vi "publishSlitWidth.vi"(8 "error in (no error)":errorcluster, 10 "slitPosition":T1, 11 "Monochromator in":refnum<class "Monochromator.lvclass">) -> (0 "error out":errorcluster, 3 "Monochromator out":refnum<class "Monochromator.lvclass">)   [LabVIEW 2016, in "Monochromator.lvclass"]
uses:
  Monochromator.lvclass
  Typedefs/slit.ctl
  Typedefs/SlitType.ctl
  Typedefs/slitWidth.ctl
  Monochromator.lvclass/Monochromator.ctl
  MonoPubSubData/MonoPubSubData.lvclass/MonoPubSubData.ctl
  MonoPubSubData/MonoPubSubData.lvclass
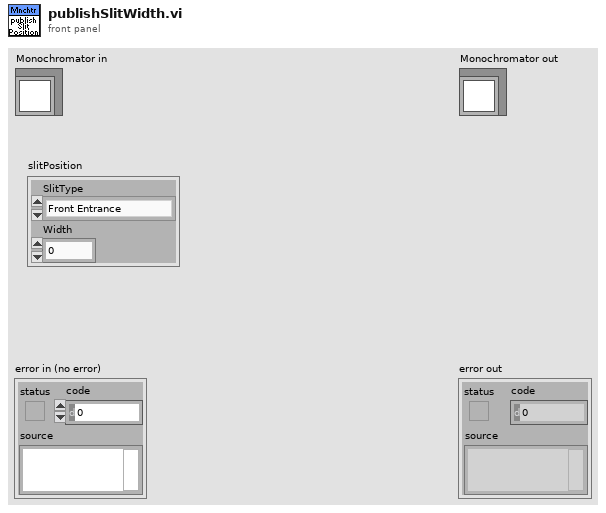
[diagram p1: front panel]
types:
  T1 = typedef "slit.ctl" = cluster{"SlitType":T2, "Width":T3}
  T2 = typedef "SlitType.ctl" = enum16{"Front Entrance", "Side Entrance", "Front Exit", "Side Exit", "First Intermediate", "Second Intermediate"}
  T3 = typedef "slitWidth.ctl" = dbl
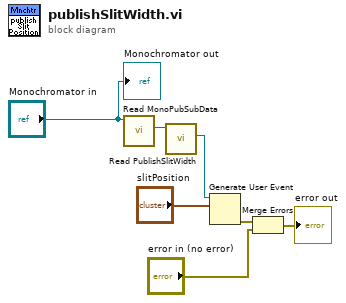
[diagram p0: block diagram]
diagram:
  n1 = call "Read MonoPubSubData.vi"("Monochromator in"="Monochromator in") -> ("MonoPubSubData.lvclass"=w4:refnum<class "MonoPubSubData.lvclass">)  [unwired: 8 in, 2 out]
  n2 = call "Read PublishSlitWidth.vi"("MonoPubSubData in"=w4) -> ("PublishSlitPosition"=w5:refnum<user-event>)  [unwired: 8 in, 2 out]
  n3 = Generate User Event(user event=w5, event data cluster="slitPosition") -> (error out=w3:errorcluster)  [unwired: 2 in, 1 out]
  n4 = Merge Errors(w3, "error in (no error)") -> (→"error out":errorcluster)
  "Monochromator out" <- "Monochromator in"
